vi "Write Pulse duration.vi"(10 "Pulse duration (ms)":u32=50, 11 "TTL in":refnum<class "TTL.lvclass">) -> (3 "TTL out":refnum<class "TTL.lvclass">)   [LabVIEW 2011, in "TTL.lvclass"]
uses:
  TTL.lvclass
  TTL.lvclass/TTL.ctl
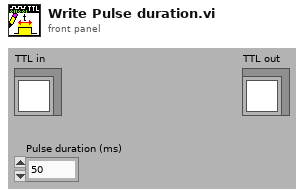
[diagram p1: front panel]
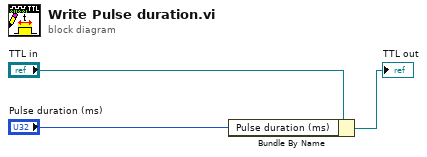
[diagram p0: block diagram]
diagram:
  n1 = Bundle By Name(cluster="TTL in", "Pulse duration (ms)"="Pulse duration (ms)") -> (→"TTL out":refnum<class "TTL.lvclass">)
